vi "求导曲率半径.vi"(9 "x":dbl[](array[numeric]), 10 "y":dbl[](array[numeric])) -> (1 "x/y":dbl[](array[numeric]), 2 "?":cluster{"Data_x":dbl[], "Data_y":dbl[]}(graph))   [LabVIEW 2016]
uses:
  <vilib>/express/express arith-compare/Formula/XNode/ExpressFormulaBlockNode.xnode
  <vilib>/Analysis/NI_AALPro.lvlib
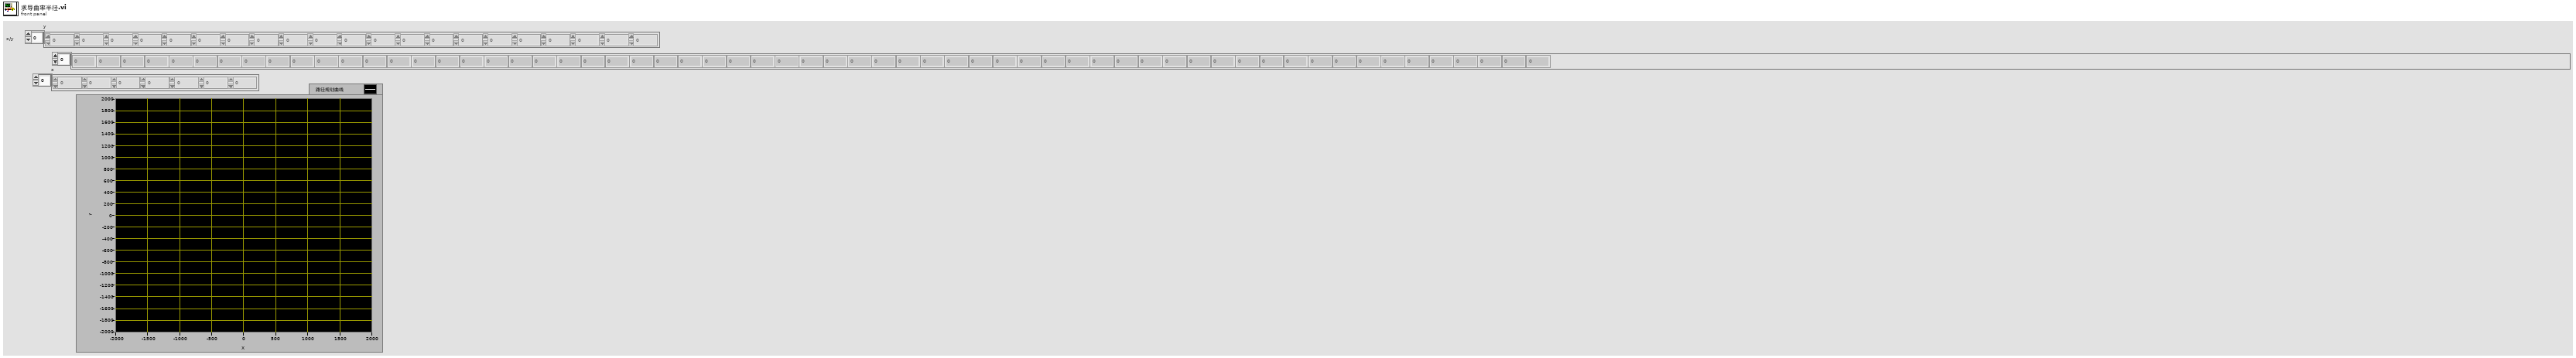
[diagram p1: front panel]
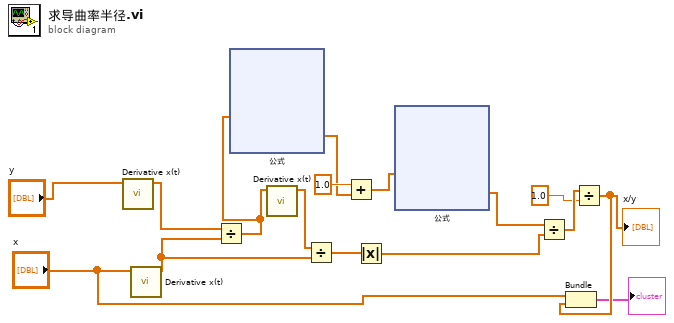
[diagram p0: block diagram]
diagram:
  n1 = call <vilib>:"Derivative x(t).vi"("X"="y") -> ("dX/dt"=w1:dbl[])  [unwired: 9 in, 1 out]
  n2 = call <vilib>:"Derivative x(t).vi"("X"="x") -> ("dX/dt"=w10:dbl[])  [unwired: 9 in, 1 out]
  n3 = Divide(x=w1, y=w10) -> (x/y=w8:dbl[])
  n4 = xnode "公式"("X1"=w8) -> ("结果"=w7:dbl[])  [unwired: 1 in, 1 out]
  n5 = call <vilib>:"Derivative x(t).vi"("X"=w8) -> ("dX/dt"=w11:dbl[])  [unwired: 9 in, 1 out]
  n6 = Divide(x=w11, y=w10) -> (x/y=w16:dbl[])
  n7 = Add(x=1.0, y=w7) -> (x+y=w14:dbl[])
  n8 = Absolute Value(x=w16) -> (abs(x)=w12:dbl[])
  n9 = xnode "公式"("X1"=w14) -> ("结果"=w13:dbl[])  [unwired: 1 in, 1 out]
  n10 = Divide(x=w13, y=w12) -> (x/y=w6:dbl[])
  n11 = Divide(x=w6, y=1.0 ("x")) -> (x/y=w4:dbl[])
  "x/y" <- w4
  n12 = Bundle("x"="x", w4) -> (→"?":cluster{"x":dbl[], dbl[]})  [unwired: 1 in]
